vi "LVClass_WavefrontCorrector Write WavefrontCorrector.vi"(8 "error in (no error)":errorcluster, 10 "WavefrontCorrector":i32, 11 "WavefrontCorrector in":refnum<class "WavefrontCorrector.lvclass">) -> (0 "error out":errorcluster, 3 "WavefrontCorrector out":refnum<class "WavefrontCorrector.lvclass">)   [LabVIEW 2020, in "WavefrontCorrector.lvclass"]
uses:
  WavefrontCorrector.lvclass
  WavefrontCorrector.lvclass/WavefrontCorrector.ctl
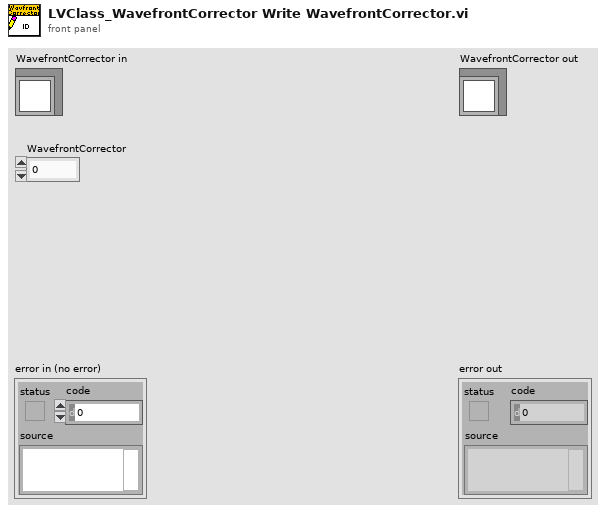
[diagram p1: front panel]
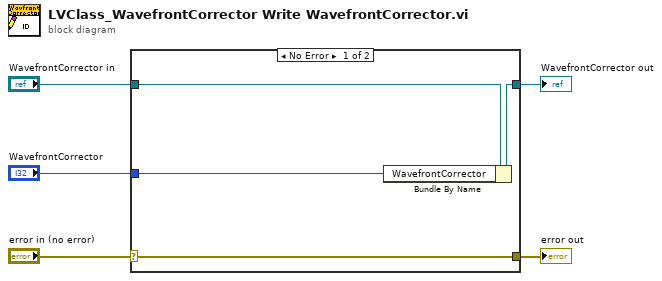
[diagram p0: block diagram]
diagram:
  n1 = case shown="No Error" "error in (no error)" {
    selector: "error in (no error)" -> [w9 w10]
    tunnel: [w9 w10] -> w4
    tunnel: [w7 w11] -> w2
    tunnel: "WavefrontCorrector in" -> [w8 w11]
    tunnel: "WavefrontCorrector" -> [w6 _]
    frame No Error {
      n2 = Bundle By Name(cluster=w8, "WavefrontCorrector"=w6) -> (w7:refnum<class "WavefrontCorrector.lvclass">)
    }
    frame Error {
    }
  }
  "error out" <- w4
  "WavefrontCorrector out" <- w2
